vi "Get measurement coordinates.vi"(5 "Trap cluster":T1, 6 "Switch xy":bool, 7 "Coordinate mapping \n(Monitor to Measurement)":T2) -> (0 "X (Measurement)":sgl[](array[numeric]), 1 "Y (Measurement)":sgl[](array[numeric]))   [LabVIEW 2012]
uses:
  Trap cluster.ctl
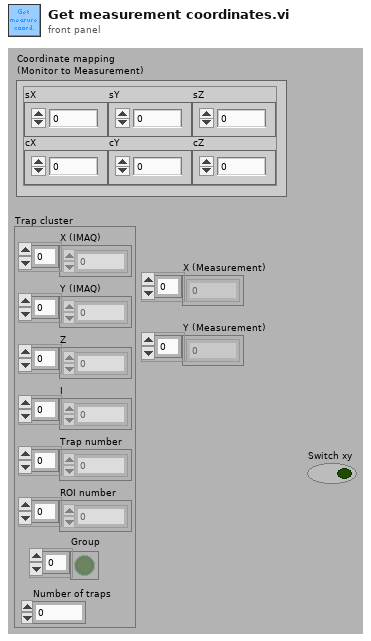
[diagram p1: front panel]
types:
  T1 = typedef "Trap cluster.ctl" = cluster{"X (IMAQ)":sgl[], "Y (IMAQ)":sgl[], "Z":sgl[], "I":sgl[], "Trap number":i32[], "ROI number":i32[], "Number of traps":i32, "Group":bool[]}
  T2 = cluster{"cZ":sgl, "cY":sgl, "cX":sgl, "sZ":sgl, "sY":sgl, "sX":sgl}
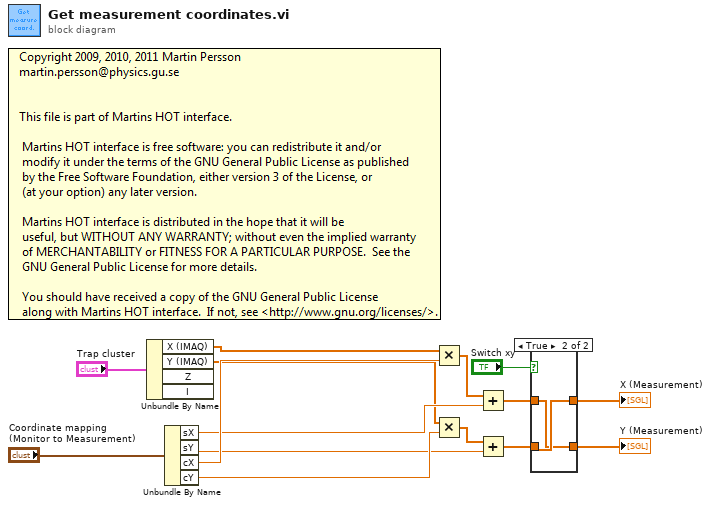
[diagram p0: block diagram]
diagram:
  n1 = Unbundle By Name("Trap cluster") -> ("X (IMAQ)"=w8:sgl[], "Y (IMAQ)"=w7:sgl[])  [unwired: 2 out]
  n2 = Unbundle By Name("Coordinate mapping \n(Monitor to Measurement)") -> ("sX"=w12:sgl, "sY"=w13:sgl, "cX"=w14:sgl, "cY"=w15:sgl)
  n3 = Multiply(x=w8, y=w14) -> (x*y=w10:sgl[])
  n4 = Multiply(x=w7, y=w15) -> (x*y=w11:sgl[])
  n5 = Add(x=w10, y=w12) -> (x+y=w4:sgl[])
  n6 = Add(x=w11, y=w13) -> (x+y=w3:sgl[])
  n7 = case shown="True" "Switch xy" {
    tunnel: w4 -> [w17 w18]
    tunnel: w3 -> [w16 w19]
    tunnel: [w17 w19] -> w2
    tunnel: [w16 w18] -> w1
    frame False {
    }
    frame True {
    }
  }
  "X (Measurement)" <- w2
  "Y (Measurement)" <- w1
